vi "Subpanel - Latch Test.vi"(0 "VI Reference In":refnum<vi>, 5 "Subpanel Details":string, 11 "error in (no error)":errorcluster) -> (4 "VI Reference Out":refnum<vi>, 15 "error out":errorcluster)   [LabVIEW 2016]
uses:
  APIs/Stimulus/ControlValue/ValueSignalLatchBooleanString.vi
  APIs/Assert/AssertControlValue/Equal.vi
  <vilib>/addons/_JKI Toolkits/Caraya/classes/Test/Test.lvclass
  Drona.lvlib
  apis/Assert/AssertControlValue/AssertControlValue.lvlib
  APIs/Stimulus/ValueSignal/ControlValue.lvlib
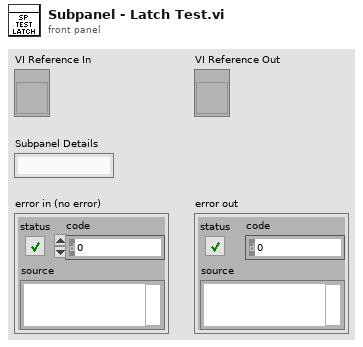
[diagram p1: front panel]
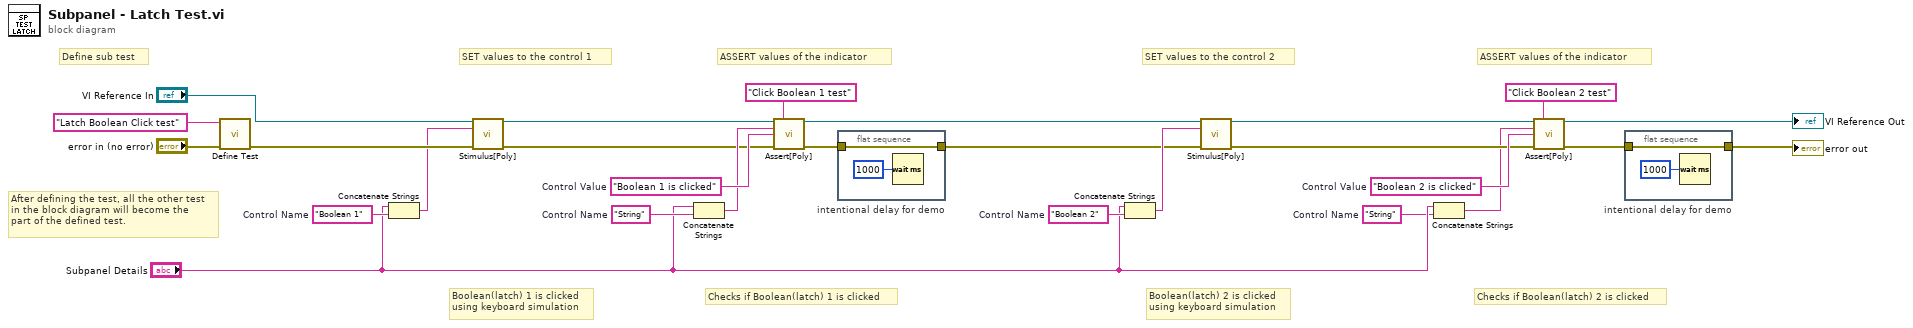
[diagram p0: block diagram]
diagram:
  w7 = "String"  # Control Name
  w22 = "Boolean 2 is clicked"  # Control Value
  w10 = "Boolean 2"  # Control Name
  w12 = "String"  # Control Name
  w25 = "Boolean 1 is clicked"  # Control Value
  w14 = "Boolean 1"  # Control Name
  # "Checks if Boolean(latch) 2 is clicked"
  # "ASSERT values of the indicator"
  # "Boolean(latch) 2 is clicked\nusing keyboard simulation"
  # "SET values to the control 2"
  # "Checks if Boolean(latch) 1 is clicked"
  # "ASSERT values of the indicator"
  # "Boolean(latch) 1 is clicked\nusing keyboard simulation"
  # "SET values to the control 1"
  # "After defining the test, all the other test\nin the block diagram will become the \npart of the defined test."
  # "Define sub test"
  n1 = call <vilib>:"Define Test.vi"("error in (no error)"="error in (no error)", "Label (VI Title)"="Latch Boolean Click test") -> ("error out"=w18:errorcluster)  [unwired: 9 in]
  n2 = Concatenate Strings("Subpanel Details", w14) -> (w13:string)
  n3 = call-poly "Stimulus[Poly].vi"("VI Reference In"="VI Reference In", "Control Path"=w13, "error in"=w18) -> ("VI Reference Out"=w26:refnum<vi>, "error out"=w5:errorcluster)  [unwired: 11 in]
  n4 = Concatenate Strings("Subpanel Details", w12) -> (w11:string)
  n5 = call-poly "Assert[Poly].vi"("VI Reference In"=w26, "Label"="Click Boolean 1 test" ("Label (VI Title)"), "Control Path"=w11, "Control Value"=w25, "Error In"=w5) -> ("VI Reference Out"=w21:refnum<vi>, "Error Out"=w4:errorcluster)  [unwired: 9 in]
  n6 = flat-sequence "intentional delay for demo" {
    tunnel: w4 -> [w28]
    tunnel: [w28] -> w3
    frame #0 {
      n7 = Wait (ms)(milliseconds to wait=u32 1000) -> ()  [unwired: 1 out]
    }
  }
  n8 = Concatenate Strings("Subpanel Details", w10) -> (w9:string)
  n9 = call-poly "Stimulus[Poly].vi"("VI Reference In"=w21, "Control Path"=w9, "error in"=w3) -> ("VI Reference Out"=w19:refnum<vi>, "error out"=w20:errorcluster)  [unwired: 11 in]
  n10 = Concatenate Strings("Subpanel Details", w7) -> (w6:string)
  n11 = call-poly "Assert[Poly].vi"("VI Reference In"=w19, "Label"="Click Boolean 2 test" ("Label (VI Title)"), "Control Path"=w6, "Control Value"=w22, "Error In"=w20) -> ("VI Reference Out"=→"VI Reference Out":refnum<vi>, "Error Out"=w2:errorcluster)  [unwired: 9 in]
  n12 = flat-sequence "intentional delay for demo" {
    tunnel: w2 -> [w30]
    tunnel: [w30] -> w1
    frame #0 {
      n13 = Wait (ms)(milliseconds to wait=u32 1000) -> ()  [unwired: 1 out]
    }
  }
  "error out" <- w1
